vi "Replace GUIDs in Custom Device XML.vi"(7 "error in":errorcluster, 9 "guid map":map{string, string}(c390), 10 "CustomDevice in":refnum<k24>) -> (0 "error out":errorcluster, 3 "CustomDevice out":refnum<k24>)   [LabVIEW 2020, in "Utility.lvlib"]
uses:
  Utility.lvlib
  NationalInstruments.VeriStand.XMLReader
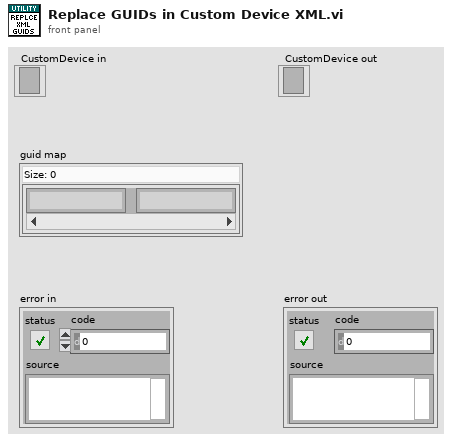
[diagram p1: front panel]
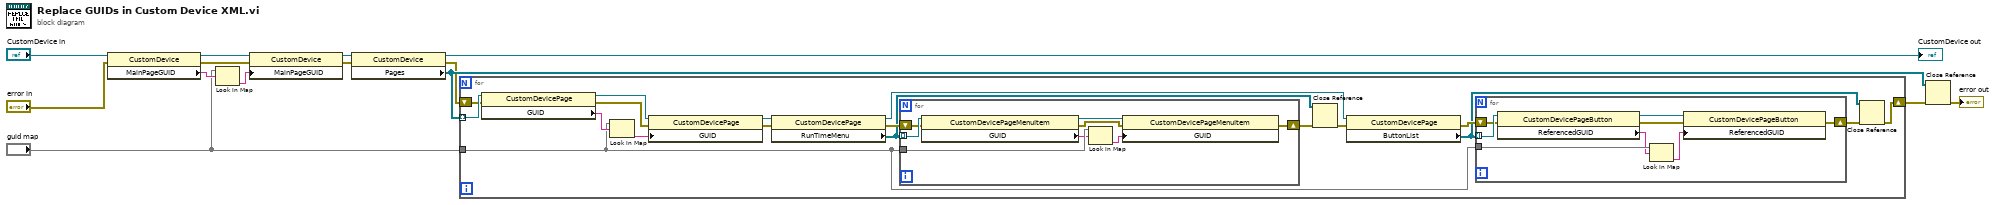
[diagram p0: block diagram]
diagram:
  n1 = property class="CustomDevice"(reference="CustomDevice in", error in="error in") -> (reference out=w11:refnum<k24>, error out=w3:errorcluster, "MainPageGUID"=w12:string)
  n2 = Look In Map(map="guid map", key=w12) -> (value=w9:string)  [unwired: 1 in, 1 out]
  n3 = property class="CustomDevice"(reference=w11, error in=w3, "MainPageGUID"=w9) -> (reference out=w10:refnum<k24>, error out=w4:errorcluster)
  n4 = property class="CustomDevice"(reference=w10, error in=w4) -> (reference out=→"CustomDevice out":refnum<k24>, error out=w5:errorcluster, "Pages"=w6:refnum<k24>[])
  n5 = for {
    tunnel: w6 -> [w32] mode=indexing
    tunnel: "guid map" -> [w26]
    shift-right: [w18] -> w7
    shift-left: w5 -> [w17]
    n6 = property class="CustomDevicePage"(reference=w32, error in=w17) -> (reference out=w29:refnum<k24>, error out=w16:errorcluster, "GUID"=w30:string)
    n7 = Look In Map(map=w26, key=w30) -> (value=w27:string)  [unwired: 1 in, 1 out]
    n8 = property class="CustomDevicePage"(reference=w29, error in=w16, "GUID"=w27) -> (reference out=w28:refnum<k24>, error out=w15:errorcluster)
    n9 = property class="CustomDevicePage"(reference=w28, error in=w15) -> (reference out=w31:refnum<k24>, error out=w23:errorcluster, "RunTimeMenu"=w20:refnum<k24>[])
    n10 = for {
      tunnel: w20 -> [w48] mode=indexing
      tunnel: w26 -> [w46]
      shift-right: [w42] -> w21
      shift-left: w23 -> [w43]
      n11 = property class="CustomDevicePageMenuItem"(reference=w48, error in=w43) -> (reference out=w47:refnum<k24>, error out=w41:errorcluster, "GUID"=w45:string)
      n12 = Look In Map(map=w46, key=w45) -> (value=w44:string)  [unwired: 1 in, 1 out]
      n13 = property class="CustomDevicePageMenuItem"(reference=w47, error in=w41, "GUID"=w44) -> (error out=w42:errorcluster)  [unwired: 1 out]
    }
    n14 = Close Reference(reference=w20, error in (no error)=w21) -> (error out=w19:errorcluster)
    n15 = property class="CustomDevicePage"(reference=w31, error in=w19) -> (error out=w24:errorcluster, "ButtonList"=w22:refnum<k24>[])  [unwired: 1 out]
    n16 = for {
      tunnel: w22 -> [w40] mode=indexing
      tunnel: w26 -> [w39]
      shift-right: [w35] -> w25
      shift-left: w24 -> [w34]
      n17 = property class="CustomDevicePageButton"(reference=w40, error in=w34) -> (reference out=w36:refnum<k24>, error out=w33:errorcluster, "ReferencedGUID"=w38:string)
      n18 = Look In Map(map=w39, key=w38) -> (value=w37:string)  [unwired: 1 in, 1 out]
      n19 = property class="CustomDevicePageButton"(reference=w36, error in=w33, "ReferencedGUID"=w37) -> (error out=w35:errorcluster)  [unwired: 1 out]
    }
    n20 = Close Reference(reference=w22, error in (no error)=w25) -> (error out=w18:errorcluster)
  }
  n21 = Close Reference(reference=w6, error in (no error)=w7) -> (error out=→"error out":errorcluster)
